vi "Stop Core.vi"(10 "final error code":i32, 11 "ATM Controller in":refnum<class "ATM Controller.lvclass">) -> (3 "ATM Controller out":refnum<class "ATM Controller.lvclass">)   [LabVIEW 2019, in "ATM Controller.lvlib" / "ATM Controller.lvclass"]
doc: "(<B>Filename</B>: Actor Framework.lvlib:Actor.lvclass:Stop Core.vi)\n\nDefines what the actor does before it stops. Use the <B>final error code</B> input to determine whether the actor shut down in response to an error.\n\nBy default, this method passes the Stop message along to all auto-stop nested actors. A descendant class may override this method to define additional behavior, such as shutting down any processes the actor initiated in its override of the Actor Core method."
uses:
  ATM Controller.lvclass
  ATM Controller.lvclass/ATM Controller.ctl
  <vilib>/ActorFramework/Actor/Actor.lvclass
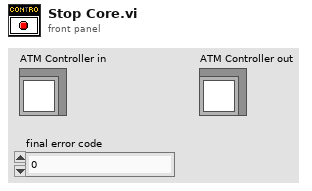
[diagram p1: front panel]
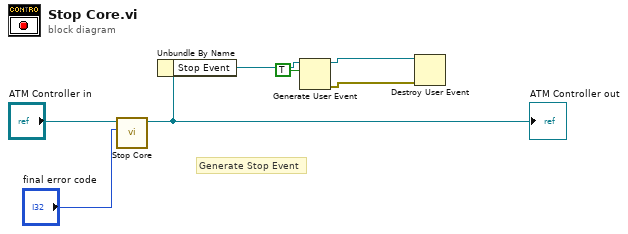
[diagram p0: block diagram]
diagram:
  # "Generate Stop Event"
  n1 = call-parent "Stop Core.vi"("final error code"="final error code", "Actor in"="ATM Controller in") -> ("Actor out"=w3:refnum<class "ATM Controller.lvclass">)  [unwired: 9 in]
  "ATM Controller out" <- w3
  n2 = Unbundle By Name(w3) -> ("Stop Event"=w2:refnum<user-event>)
  n3 = Generate User Event(user event=w2, event data cluster=TRUE ("event data")) -> (user event out=w4:refnum<user-event>, error out=w5:errorcluster)  [unwired: 2 in]
  n4 = Destroy User Event(user event=w4, error in=w5) -> ()  [unwired: 1 out]
